vi "makewave_DMD.vi"() -> ()   [LabVIEW 2012]
uses:
  <vilib>/Waveform/DWDTOps.llb/DWDT Boolean Array to Digital.vi
panel:
  in  "Stop program":bool
  in  "Add Peak":bool
  out "Digital Waveform Graph":digitalwaveform(graph)
  in  "Number of Waveforms":i32
  out "Matlab error":errorcluster
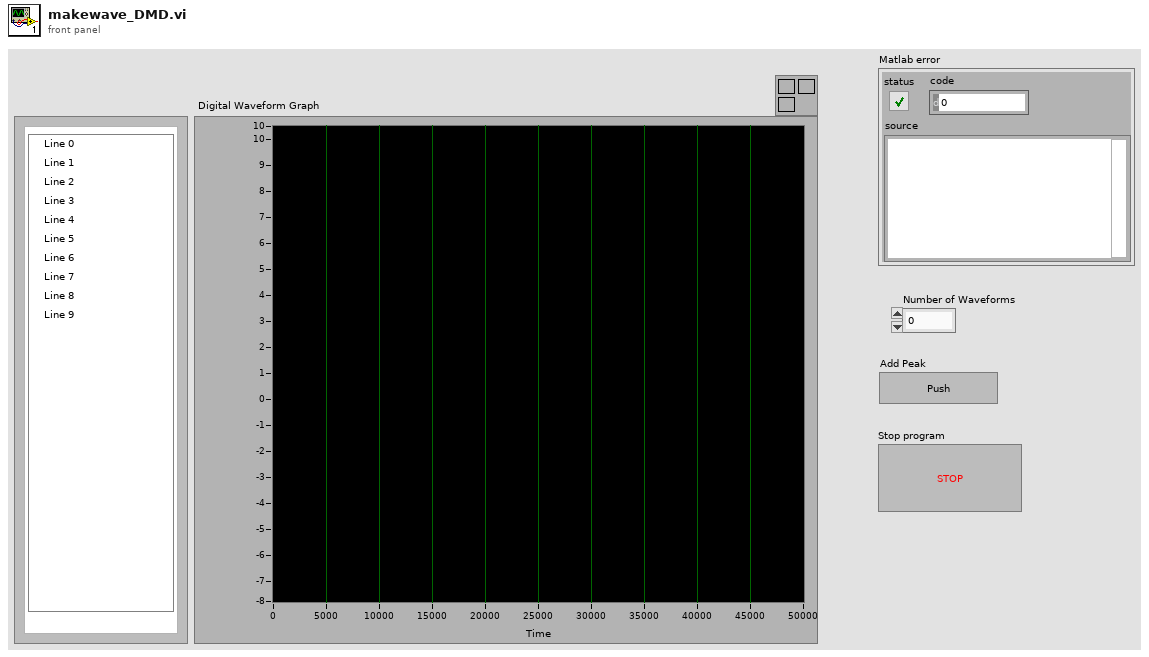
[diagram p1: front panel]
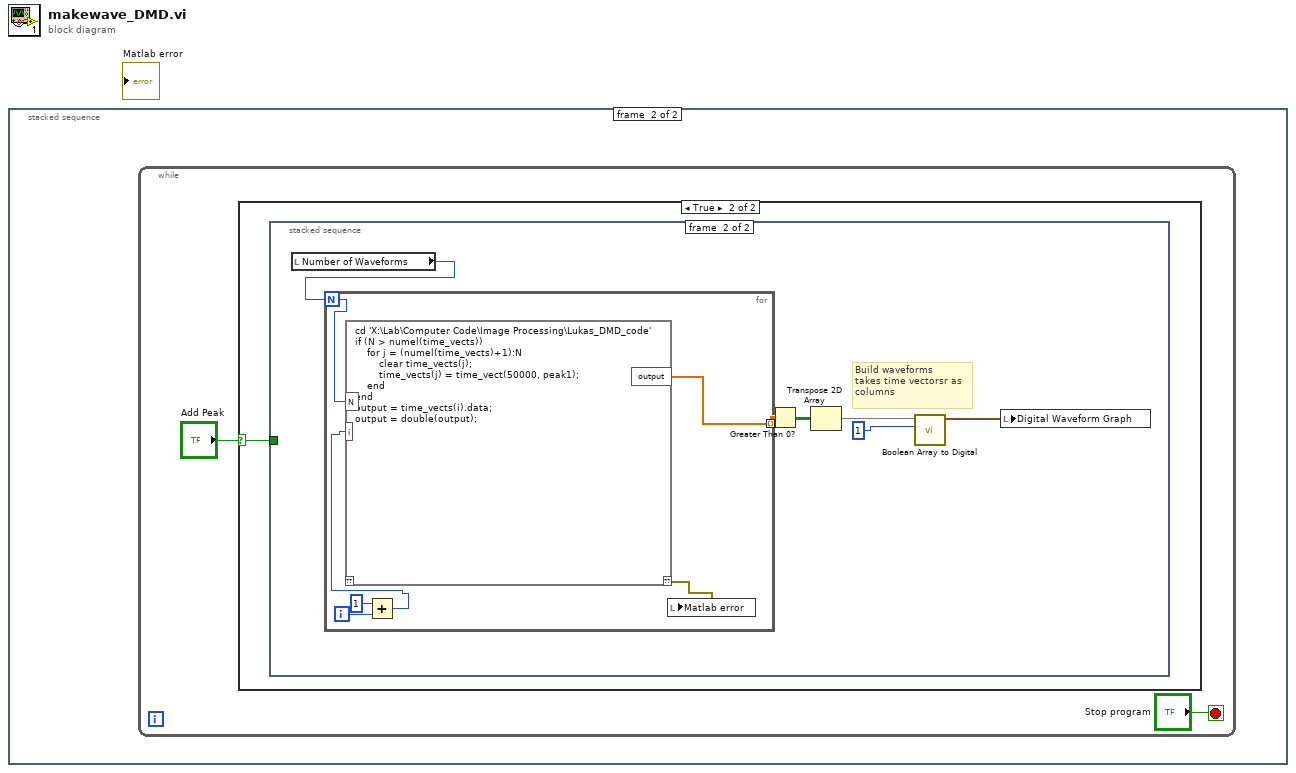
[diagram p0: block diagram]
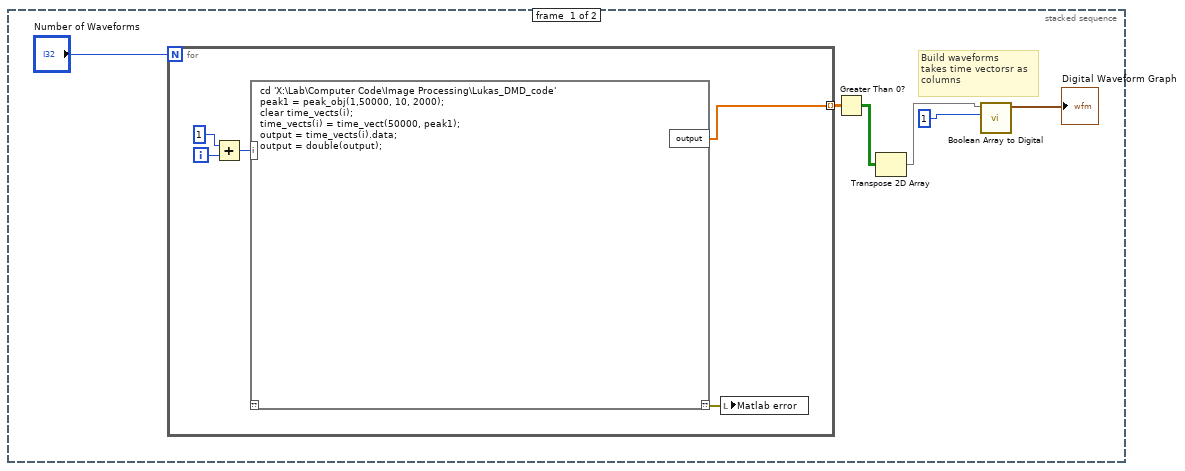
[diagram p2: hidden frame]
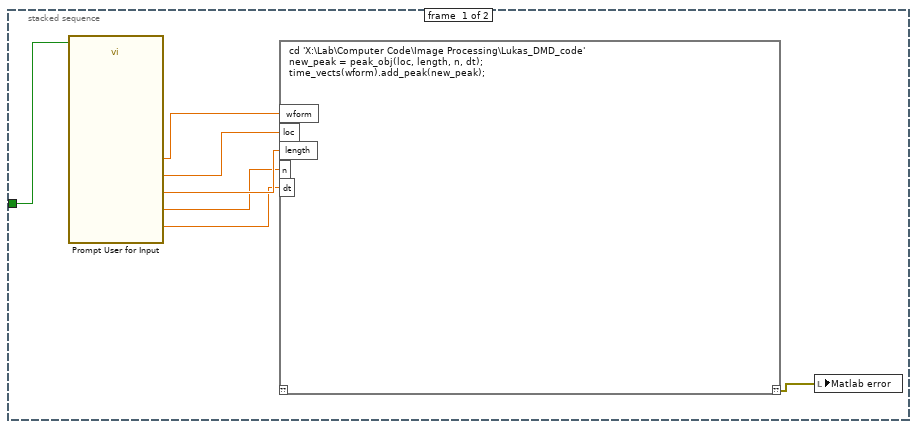
[diagram p4: hidden frame]
diagram:
  n1 = stacked-sequence {
    frame #0 {
      # "Build waveforms\ntakes time vectorsr as \ncolumns"
      n2 = for {
        N: "Number of Waveforms" -> [_]
        tunnel: [w7] -> w6 mode=indexing
        i -> [w11]
        n3 = Add(x=1, y=w11) -> (x+y=w9:i32)
        n4 = script code="cd 'X:\\Lab\\Computer Code\\Image Processing\\Lukas_DMD_code'\npeak1 = peak_obj(1,50000, 10, 2000);\nclear time_vects(i); \ntime_vects(i) = time_vect(50000, peak1); \noutput = time_vects(i).data; \noutput = double(output);"("i"=w9) -> ("??"=w8:errorcluster, "output"=w7:dbl[])  [unwired: 1 in]
        n5 = local write "Matlab error"(w8) -> ()
      }
      n6 = Greater Than 0?(x=w6) -> (x > 0?=w2:bool[][])
      n7 = Transpose 2D Array(2D array=w2) -> (transposed array=w1:bool[][])
      n8 = call-poly <vilib>:"Boolean Array to Digital.vi"("sample rate"=1, "boolean array"=w1) -> ("digital waveform"=→"Digital Waveform Graph":digitalwaveform)  [unwired: 3 in, 6 out]
    }
    frame #1 {
      n9 = while {
        stop <- "Stop program" stop-if-true
        n10 = case shown="True" "Add Peak" {
          selector: "Add Peak" -> [_ w14]
          frame False {
          }
          frame True {
            n11 = stacked-sequence {
              tunnel: w14 -> [w15 _]
              frame #0 {
                n12 = call "Prompt User for Input"("Enable"=w15) -> ("Length of each pulse:"=w16:dbl, "Number of Pulses:"=w17:dbl, "Length of Peak:"=w18:dbl, "Start of Peak:"=w19:dbl, "Which waveform:"=w20:dbl)  [unwired: 12 in, 2 out]
                n13 = script code="cd 'X:\\Lab\\Computer Code\\Image Processing\\Lukas_DMD_code'\nnew_peak = peak_obj(loc, length, n, dt); \ntime_vects(wform).add_peak(new_peak);"("wform"=w20, "loc"=w19, "length"=w18, "n"=w17, "dt"=w16) -> ("??"=w21:errorcluster)  [unwired: 1 in]
                n14 = local write "Matlab error"(w21) -> ()
              }
              frame #1 {
                # "Build waveforms\ntakes time vectorsr as \ncolumns"
                n15 = local read "Number of Waveforms"() -> (w25:i32)
                n16 = for {
                  N: w25 -> [w28]
                  tunnel: [w33] -> w23 mode=indexing
                  i -> [w31]
                  n17 = Add(x=1, y=w31) -> (x+y=w29:i32)
                  n18 = script code="cd 'X:\\Lab\\Computer Code\\Image Processing\\Lukas_DMD_code'\nif (N > numel(time_vects))\n    for j = (numel(time_vects)+1):N\n        clear time_vects(j); \n        time_vects(j) = time_vect(50000, peak1); \n    end\nend \noutput = time_vects(i).data; \noutput = double(output);"("i"=w29, "N"=w28) -> ("??"=w32:errorcluster, "output"=w33:dbl[])  [unwired: 1 in]
                  n19 = local write "Matlab error"(w32) -> ()
                }
                n20 = Greater Than 0?(x=w23) -> (x > 0?=w22:bool[][])
                n21 = Transpose 2D Array(2D array=w22) -> (transposed array=w24:bool[][])
                n22 = call-poly <vilib>:"Boolean Array to Digital.vi"("sample rate"=1, "boolean array"=w24) -> ("digital waveform"=w26:digitalwaveform)  [unwired: 3 in, 6 out]
                n23 = local write "Digital Waveform Graph"(w26) -> ()
              }
            }
          }
        }
      }
    }
  }
